vi "abortDriver_Feng.vi"(10 "litho comm":T1) -> ()   [LabVIEW 2013]
uses:
  Global Variables.vi
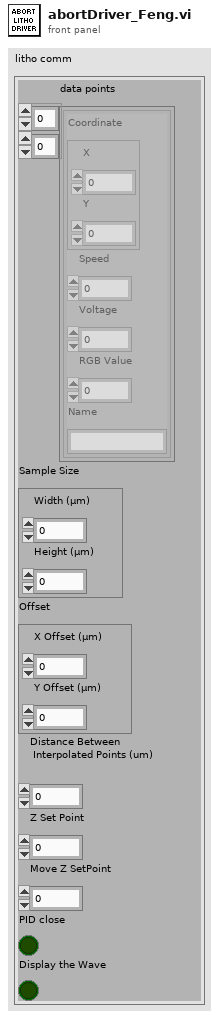
[diagram p1: front panel]
types:
  T1 = cluster{"data points":cluster{"Coordinate":cluster{"X":dbl, "Y":dbl}, "Speed":dbl, "Voltage":dbl, "RGB Value":i32, "Name":string}[][], "Sample Size":cluster{"Width (µm)":dbl, "Height (µm)":dbl}, "Offset":cluster{"X Offset (µm)":dbl, "Y Offset (µm)":dbl}, "Distance Between\n Interpolated Points (um)":dbl, "Z Set Point":dbl, "Move Z SetPoint":dbl, "PID close":bool, "Display the Wave":bool}
  T2 = cluster{"Coordinate":cluster{"X":dbl, "Y":dbl}, "Speed":dbl, "Voltage":dbl, "RGB Value":i32, "Name":string}[][]
  T3 = cluster{"X Offset (µm)":dbl, "Y Offset (µm)":dbl}
  T4 = cluster{"Coordinate":cluster{"X":dbl, "Y":dbl}, "Speed":dbl, "Voltage":dbl, "RGB Value":i32, "Name":string}
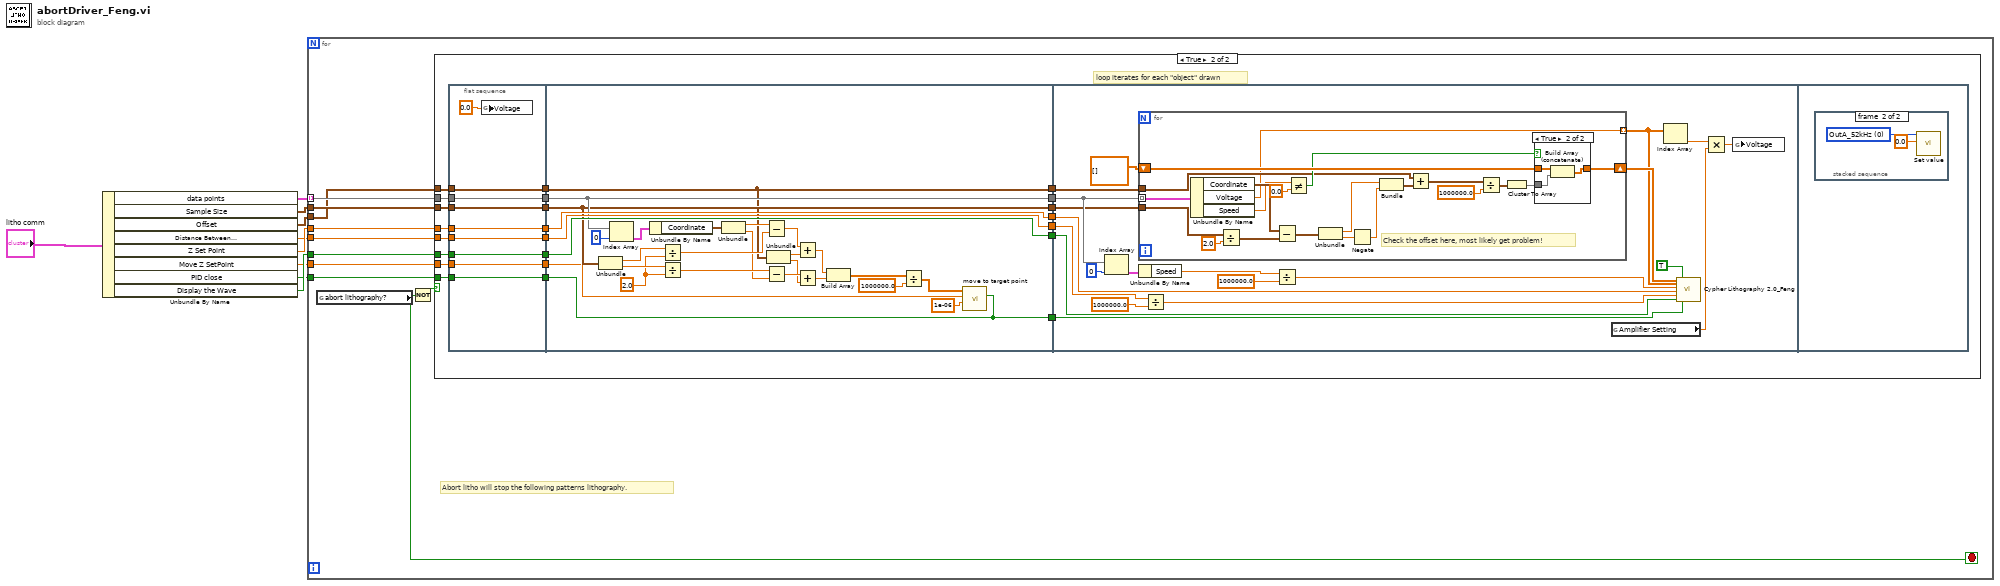
[diagram p0: block diagram]
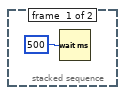
[diagram p4: hidden frame]
diagram:
  n1 = Unbundle By Name("litho comm") -> ("data points"=w2:T2, "Sample Size"=w3:cluster{"Width (µm)":dbl, "Height (µm)":dbl}, "Offset"=w4:T3, "Distance Between\n Interpolated Points (um)"=w5:dbl, "Z Set Point"=w6:dbl, "Move Z SetPoint"=w7:dbl, "PID close"=w8:bool, "Display the Wave"=w9:bool)
  n2 = for {
    tunnel: w5 -> [w14]
    tunnel: w2 -> [w19] mode=indexing
    tunnel: w6 -> [w18]
    tunnel: w9 -> [w17]
    tunnel: w8 -> [w16]
    tunnel: w3 -> [w15]
    tunnel: w4 -> [w13]
    tunnel: w7 -> [w12]
    stop <- w10 stop-if-true
    # "Abort litho will stop the following patterns lithography."
    n3 = global read "Global Variables.vi" "abort lithography?"() -> (w10:bool)
    n4 = Not(x=w10) -> (.not. x?=w11:bool)
    n5 = case shown="True" w11 {
      tunnel: w19 -> [_ w27]
      tunnel: w18 -> [_ w26]
      tunnel: w17 -> [_ w25]
      tunnel: w16 -> [_ w24]
      tunnel: w15 -> [_ w23]
      tunnel: w14 -> [_ w22]
      tunnel: w13 -> [_ w21]
      tunnel: w12 -> [_ w20]
      frame False {
      }
      frame True {
        # "loop iterates for each \"object\" drawn"
        n6 = flat-sequence {
          tunnel: w21 -> [w45]
          tunnel: w22 -> [w46]
          tunnel: w23 -> [w47]
          tunnel: w24 -> [w48]
          tunnel: w25 -> [w49]
          tunnel: w26 -> [w50]
          tunnel: w27 -> [w51]
          tunnel: [w51] -> w42
          tunnel: [w50] -> w41
          tunnel: [w49] -> w40
          tunnel: [w48] -> w39
          tunnel: [w47] -> w38
          tunnel: [w46] -> w37
          tunnel: [w45] -> w36
          tunnel: [w43] -> w35
          tunnel: w20 -> [w43]
          tunnel: [w56] -> w34
          tunnel: [w79] -> w33
          tunnel: [w78] -> w32
          tunnel: [w53] -> w31
          tunnel: [w55] -> w30
          tunnel: [w77] -> w29
          tunnel: [w54] -> w28
          tunnel: w42 -> [w56]
          tunnel: w41 -> [w79]
          tunnel: w40 -> [w78]
          tunnel: w39 -> [w53]
          tunnel: w38 -> [w55]
          tunnel: w37 -> [w77]
          tunnel: w36 -> [w54]
          tunnel: w35 -> [w52]
          tunnel: w34 -> [w100]
          tunnel: w33 -> [w85]
          tunnel: w32 -> [w87]
          tunnel: w31 -> [w88]
          tunnel: w30 -> [w97]
          tunnel: w29 -> [w93]
          tunnel: w28 -> [w91]
          frame #0 {
            n7 = global write "Global Variables.vi" "Voltage"(0.0 ("Voltage")) -> ()
          }
          frame #1 {
            w68 = 2.0 ("y")
            n8 = Unbundle(w55) -> ("Width (µm)"=w72:dbl, "Height (µm)"=w69:dbl)
            n9 = Index Array(array=w56, index=0 ("index (row)")) -> (element=w75:T4)
            n10 = Unbundle By Name(w75) -> ("Coordinate"=w73:cluster{"X":dbl, "Y":dbl})
            n11 = Divide(x=w72, y=w68) -> (x/y=w70:dbl)
            n12 = Divide(x=w69, y=w68) -> (x/y=w67:dbl)
            n13 = Unbundle(w73) -> ("X"=w71:dbl, "Y"=w66:dbl)
            n14 = Subtract(x=w71, y=w70) -> (x-y=w65:dbl)
            n15 = Subtract(x=w67, y=w66) -> (x-y=w63:dbl)
            n16 = Unbundle(w54) -> ("X Offset (µm)"=w64:dbl, "Y Offset (µm)"=w62:dbl)
            n17 = Add(x=w65, y=w64) -> (x+y=w61:dbl)
            n18 = Add(x=w63, y=w62) -> (x+y=w60:dbl)
            n19 = Build Array(w61, w60) -> (w58:dbl[])
            n20 = Divide(x=w58, y=1000000.0) -> (x/y=w57:dbl[])
            n21 = call "move to target point.vi"("PIS Close"=w53, "Litho Speed"=1e-06, "Z SetPoint"=w52, "Target Point\n(  x      ,       y   )"=w57) -> ()  [unwired: 8 in]
          }
          frame #2 {
            n22 = Index Array(array=w100, index=0) -> (element=w98:T4)
            n23 = for {
              tunnel: w100 -> [w121] mode=indexing
              tunnel: [w101] -> w81 mode=indexing
              tunnel: w97 -> [w119]
              shift-right: [w109] -> w83
              shift-left: dbl[][] [] -> [w108]
              tunnel: w91 -> [w102]
              # "Check the offset here, most likely get problem!"
              n24 = Unbundle By Name(w121) -> ("Coordinate"=w116:cluster{"X":dbl, "Y":dbl}, "Voltage"=w101:dbl, "Speed"=w107:dbl)
              n25 = Divide(x=w119, y=2.0) -> (x/y=w115:cluster{"Width (µm)":dbl, "Height (µm)":dbl})
              n26 = Subtract(x=w116, y=w115) -> (x-y=w114:cluster{dbl, dbl})
              n27 = Not Equal?(x=w107, y=0.0) -> (x != y?=w105:bool)
              n28 = Unbundle(w114) -> (w111:dbl, w113:dbl)
              n29 = Negate(x=w113) -> (-x=w112:dbl)
              n30 = Bundle(w111, w112) -> (w104:cluster{dbl, dbl})  [unwired: 1 in]
              n31 = Add(x=w102, y=w104) -> (x+y=w103:cluster{dbl, dbl})
              n32 = Divide(x=w103, y=1000000.0) -> (x/y=w117:cluster{dbl, dbl})
              n33 = Cluster To Array(cluster=w117) -> (array=w110:dbl[])
              n34 = case shown="True" w105 {
                tunnel: w110 -> [_ w125]
                tunnel: [w122 w124] -> w109
                tunnel: w108 -> [w122 w123]
                frame False {
                }
                frame True {
                  n35 = Build Array (concatenate)(w123, w125) -> (w124:dbl[][])
                }
              }
            }
            n36 = Unbundle By Name(w98) -> ("Speed"=w95:dbl)
            n37 = Divide(x=w93, y=1000000.0) -> (x/y=w86:dbl)
            n38 = Divide(x=w95, y=1000000.0) -> (x/y=w84:dbl)
            n39 = global read "Global Variables.vi" "Amplifier Setting"() -> (w90:dbl)
            n40 = Index Array(array=w81) -> (element=w89:dbl)  [unwired: 1 in]
            n41 = call "Cypher Lithography 2.0_Feng.vi"("Nodes on the line\n(  x      ,       y   )"=w83, "V"=w81, "Litho Speed"=w84, "Z SetPoint"=w85, "New nodes spacing"=w86, "display wave"=w87, "Need interpolate new nodes?"=TRUE, "PID close"=w88) -> ()  [unwired: 12 in]
            n42 = Multiply(x=w89, y=w90) -> (x*y=w80:dbl)
            n43 = global write "Global Variables.vi" "Voltage"(w80) -> ()
          }
          frame #3 {
            n44 = stacked-sequence {
              frame #0 {
                n45 = Wait (ms)(milliseconds to wait=u32 500) -> ()  [unwired: 1 out]
              }
              frame #1 {
                w128 = u16 0 items=["OutA_52kHz", "OutB_52kHz", "OutC_78Hz", "PiezoX", "PiezoY", "PiezoZ", "DDS_Frequency1", "DDS_Frequency2", "DDS_Amplitude1", "DDS_Amplitude2", "DDS_DCOffset", "\"Setpoint%PIDSLoop.3\"", "\"Setpoint%PIDSLoop.4\"", ""] ("Output")
                n46 = call "Set value.vi"("Value"=0.0, "Output"=w128) -> ()  [unwired: 9 in, 1 out]
              }
            }
          }
        }
      }
    }
  }
